vi "Build Error String.vi"(11 "Errors":string[](array[string]) caption="错误") -> (3 "String":string caption="字符串")   [LabVIEW 2016]
panel:
  in  "Issues Message":string="请纠正以下问题：" caption="问题信息"
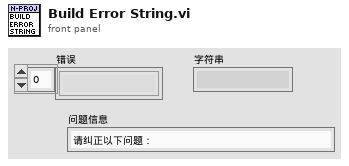
[diagram p1: front panel]
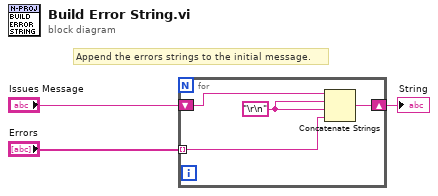
[diagram p0: block diagram]
diagram:
  # "Append the errors strings to the initial message."
  n1 = for {
    tunnel: "Errors" -> [w5] mode=indexing
    shift-right: [w6] -> w2
    shift-left: "Issues Message" -> [w7]
    w4 = "\r\n"
    n2 = Concatenate Strings(w7, w4, w4, w5) -> (w6:string)
  }
  "String" <- w2
